vi "Edgertronic-configure_camera.vi"(3 "error in (no error)":errorcluster, 4 "Settings":T1={"Frame Rate (fps)"=1000.0, "Exposure (1/sec)"=1500.0, "Horizonal"=0, "Vertical"=0, "ISO"=500, "Duration"=1.0, "Pretrigger (%)"=50.0, "MultiShot"=1, "Subsample?"=FALSE, "Force Mono?"=FALSE, "Genlock"=enum."Off", "Overclock"=enum."Off"} {"Pretrigger (%)" min=0.0 max=100.0 step=1.0; "ISO" min=0 max=1600 step=1; "Exposure (1/sec)" min=4e-06 max=250000.0 step=1.0; "Frame Rate (fps)" min=0.1 max=25000.0 step=1.0}, 5 "URL":string="130.64.17.41") -> (0 "error out":errorcluster, 1 "Saved Settings:":T3={"Requested Genlock "="20140911165611", "Min Frame Clocks "="20140911165611", "Is Seq Clk Freq "="20140911165611", "Pretrigger Frames "="20140911165611", "Duration "="20140911165611", "Overclock "="20140911165611", "Requested Horizontal "="20140911165611", "Frames "="20140911165611", "Requested Pretrigger "="20140911165611", "Words per Frame "="20140911165611", "Buffer End "="20140911165611", "Clocks per Frame  "="20140911165611", "Requested Duration "="20140911165611", "Pretrigger "="20140911165611", "Post-trigger Frames "="20140911165611", "Vertical "="20140911165611", "Requested Vertical "="20140911165611", "Reqested Frame Rate "="20140911165611", "Frame Rate "="20140911165611", "Horizontal "="20140911165611", "Clocks per Exposure "="20140911165611", "Digital Gain "="20140911165611", "Exposure "="20140911165611", "Genlock "="20140911165611", "Analog Gain "="20140911165611", "Subsample "="20140911165611", "Requested Exposure "="20140911165611", "Iso "="20140911165611", "Requested Overclock "="20140911165611", "Requested Subsample "="20140911165611", "Requested Iso"="20140911165611", "Multishot"="20140911165611", "Requested Multishot"="20140911165611", "Monochrome"="20140911165611", "Requested mono"="20140911165611", "FPGA Temp"="20140911165611", "Is Temp"="20140911165611", "Posttrigger Duration"="20140911165611", "Pretrigger Duration"="20140911165611", "dacvrefadc"="20140911165611"})   [LabVIEW 2015]
doc: "This VI configures camera settings."
uses:
  GET/SettingsCtrl.ctl
panel:
  in  "Old ConfigCamera":T2={"Requested Genlock "="0", "Requested Horizontal (pixels)"=1110.0, "Requested Duration (seconds) "=0.5, "Requested Overclock "="0", "Requested Subsample "="0", "Reqested Force Mono"="0", "Requested Vertical (pixels)"=862.0, "Reqested Frame Rate (fps)"=14687.541250000002, "Requested Exposure (seconds)"=0.08187572500000001, "Requested Pretrigger (%)"=50.0, "Requested iso"=1038.0} {"Requested iso" min=0.0 max=1600.0 step=1.0 scale=400.0..1600.0; "Requested Pretrigger (%)" min=0.0 max=100.0 step=1.0 scale=0.0..100.0; "Requested Exposure (seconds)" min=4e-06 max=0.1 step=1.0 scale=4e-06..0.1; "Reqested Frame Rate (fps)" min=0.1 max=25000.0 step=1.0 scale=0.1..25000.0; "Requested Vertical (pixels)" min=192.0 max=1280.0 step=1.0 scale=96.0..1024.0; "Requested Duration (seconds)" min=0.0; "Requested Horizontal (pixels)" min=192.0 max=1280.0 step=1.0 scale=192.0..1280.0}
  out "POST string":string="{\"requested_horizontal\": \"733\", \"requested_vertical\": \"831\", \"requested_frame_rate\": \"1000.00\", \"requested_exposure\": \"0.002000\", \"requested_duration\": \"1.00\", \"requested_pretrigger\": \"50\", \"requested_iso\": \"500\", \"requested_subsample\": \"0\", \"requested_genlock\": \"1\", \"requested_overclock\": \"0\", \"requested_force_mono\": \"0\", \"requested_multishot_count\": \"1\"}"
  in  "Configure Camera:":T4={"Duration (sec)"=1.0, "Subsample?"=FALSE, "Force Mono?"=TRUE, "Pretrigger (%)"=50.0, "ISO"=500.0, "Horizontal"=733.0, "Vertical"=831.0, "Frame Rate (fps)"=1000.0, "Genlock"=enum."Off", "Overclock"=enum."Off", "Exposure (1/sec)"=500.0, "MultiShot"=1} {"Exposure (1/sec)" min=4e-06 max=250000.0 step=1.0 scale=10.0..250000.0; "Frame Rate (fps)" min=0.1 max=25000.0 step=1.0 scale=0.1..25000.0; "Vertical" min=192.0 max=1280.0 step=1.0 scale=96.0..1024.0; "Horizontal" min=192.0 max=1280.0 step=1.0 scale=192.0..1280.0; "ISO" min=0.0 max=1600.0 step=1.0 scale=400.0..1600.0; "Pretrigger (%)" min=0.0 max=100.0 step=1.0 scale=0.0..100.0; "Duration (sec)" min=0.0}
  # "130.64.16.195"
  # "Glossary:\nHorizontal:\t(pixels)[192-1280\t]=Width of image to capture.\nVertical:\t(pixels)[96-1024]=Height of image to capture.\nFrame Rate: (frames per second)[0.1-25000]=Number of frames to capture in every second.\nExposure:(seconds)[0.000004-0.1]=Amount of time the CMOS sensor is integrating the received light.\nDuration:(seconds)[Limited by memory]=Amount of the video to capture.\nPretrigger:(percentage)[0-100]=Amount of the video being captured is captured before the trigger event.\nIso:=sensitivity to light.\n          color:[100-400]\n          mono: [400-1600] \nSubsample: =Controls skipping every other row and column.\n          0 - off\n          1 - on\t\nForce Mono\t=Force color sensor video to be processed as monochrome. This is useful for high frame rates where the de-Bayering algorithm might add noise to the image. Note: this doesn't change the \tISO range. This feature is not implemented.\n          0 - off\n          1 - on\nGenlock:\t=Camera genlock configuration. \n          0 - off \n          1 - master =Master means the camera is generating the trigger and start-of-exposure timing signals. \n          2 - slave =Slave mean the camera is receiving those signals, via the external trigger connector, from the genlock master camera.\nOverclock: =Camera overclock configuration\n          0 - off \n          1 - A level : A is the least overclocking\n          2 - B level\n          3 - C level\n          4 - D level\t : D is the most overclocking"
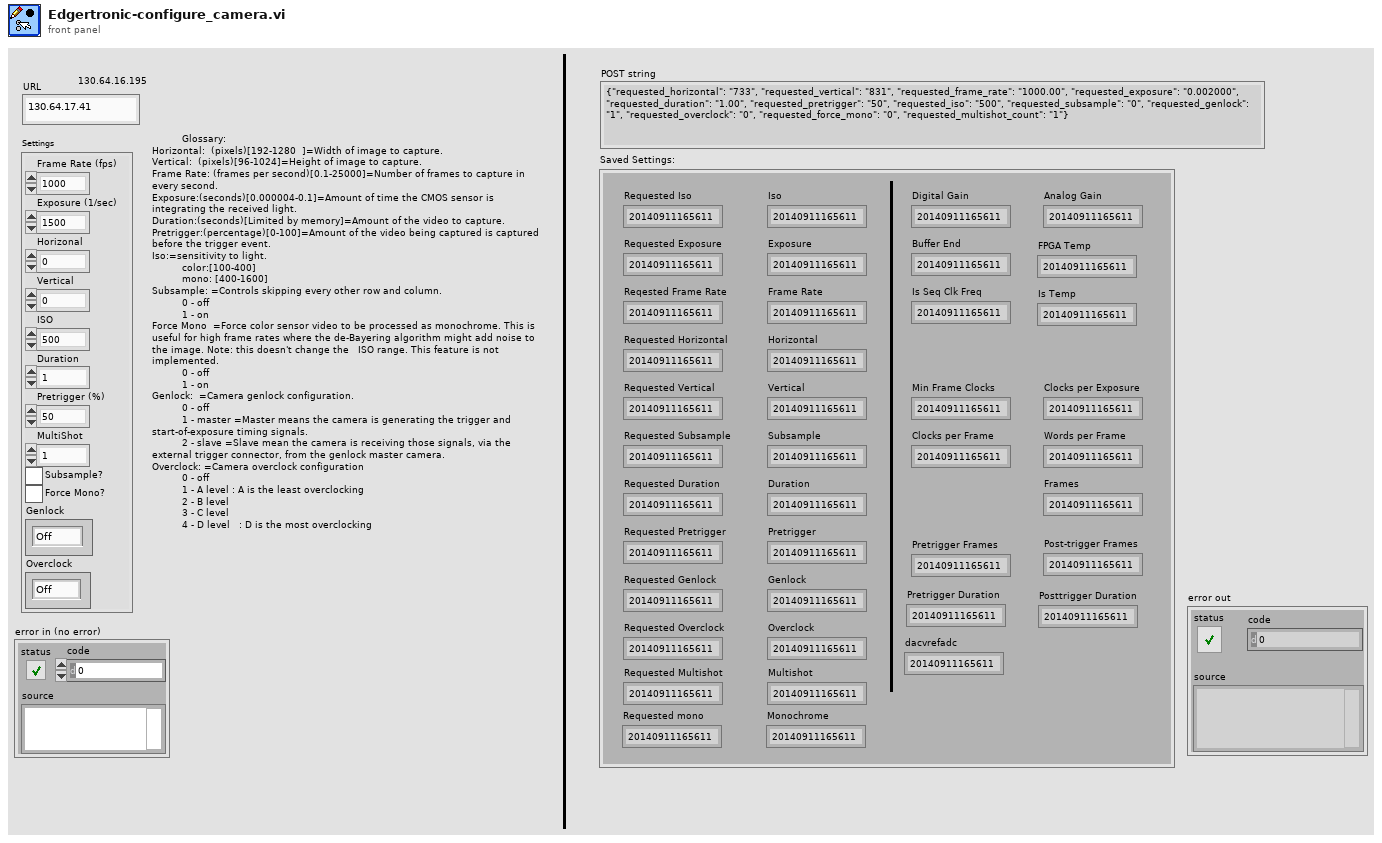
[diagram p1: front panel]
types:
  T1 = cluster{"Frame Rate (fps)":dbl, "Exposure (1/sec)":dbl, "Horizonal":u16, "Vertical":u16, "ISO":i16, "Duration":dbl, "Pretrigger (%)":dbl, "MultiShot":i16, "Subsample?":bool, "Force Mono?":bool, "Genlock":enum16{"Off", "Master", "Slave"}, "Overclock":enum16{"Off", "A level", "B Level", "C Level", "D Level"}}
  T2 = cluster{"Requested Genlock ":string, "Requested Horizontal (pixels)":dbl, "Requested Duration (seconds) ":dbl, "Requested Overclock ":string, "Requested Subsample ":string, "Reqested Force Mono":string, "Requested Vertical (pixels)":dbl, "Reqested Frame Rate (fps)":dbl, "Requested Exposure (seconds)":dbl, "Requested Pretrigger (%)":dbl, "Requested iso":dbl}
  T3 = typedef "SettingsCtrl.ctl" = cluster{"Requested Genlock ":string, "Min Frame Clocks ":string, "Is Seq Clk Freq ":string, "Pretrigger Frames ":string, "Duration ":string, "Overclock ":string, "Requested Horizontal ":string, "Frames ":string, "Requested Pretrigger ":string, "Words per Frame ":string, "Buffer End ":string, "Clocks per Frame  ":string, "Requested Duration ":string, "Pretrigger ":string, "Post-trigger Frames ":string, "Vertical ":string, "Requested Vertical ":string, "Reqested Frame Rate ":string, "Frame Rate ":string, "Horizontal ":string, "Clocks per Exposure ":string, "Digital Gain ":string, "Exposure ":string, "Genlock ":string, "Analog Gain ":string, "Subsample ":string, "Requested Exposure ":string, "Iso ":string, "Requested Overclock ":string, "Requested Subsample ":string, "Requested Iso":string, "Multishot":string, "Requested Multishot":string, "Monochrome":string, "Requested mono":string, "FPGA Temp":string, "Is Temp":string, "Posttrigger Duration":string, "Pretrigger Duration":string, "dacvrefadc":string}
  T4 = cluster{"Duration (sec)":dbl, "Subsample?":bool, "Force Mono?":bool, "Pretrigger (%)":dbl, "ISO":dbl, "Horizontal":dbl, "Vertical":dbl, "Frame Rate (fps)":dbl, "Genlock":enum16{"Off", "Master", "Slave", "External"}, "Overclock":enum16{"Off", "A level", "B Level", "C Level", "D Level"}, "Exposure (1/sec)":dbl, "MultiShot":i16}
  T5 = cluster{"Parameter":string, "Parameter 2":string, "Parameter 3":string, "Parameter 4":string, "Parameter 5":string, "Parameter 6":string, "Parameter 7":string, "Parameter 8":string, "Parameter 9":string, "Parameter 10":string, "Parameter 11":string, "Parameter 12":string}
  T6 = enum16{"Off", "A level", "B Level", "C Level", "D Level"}
  T7 = cluster{string, string, string, string, string, string, string, "output string":string, "output string":string, string, string, string}
  T8 = cluster{"Requested Genlock ":string, "Min Frame Clocks ":string, "Is Seq Clk Freq ":string, "Pretrigger Frames ":string, "Duration ":string, "Overclock ":string, "Requested Horizontal ":string, "Frames ":string, "Requested Pretrigger ":string, "Words per Frame ":string, "Buffer End ":string, "Clocks per Frame  ":string, "Requested Duration ":string, "Pretrigger ":string, "Post-trigger Frames ":string, "Vertical ":string, "Requested Vertical ":string, "Reqested Frame Rate ":string, "Frame Rate ":string, "Horizontal ":string, "Clocks per Exposure ":string, "Digital Gain ":string, "Exposure ":string, "Genlock ":string, "Analog Gain ":string, "Subsample ":string, "Requested Exposure ":string, "Iso ":string, "Requested Overclock ":string, "Requested Subsample ":string, "Requested Iso":string, "Multishot":string, "Requested Multishot":string, "Monochrome":string, "Requested mono":string, "FPGA Temp":string, "Is Temp":string, "Posttrigger Duration":string, "Pretrigger Duration":string, "dacvrefadc":string}
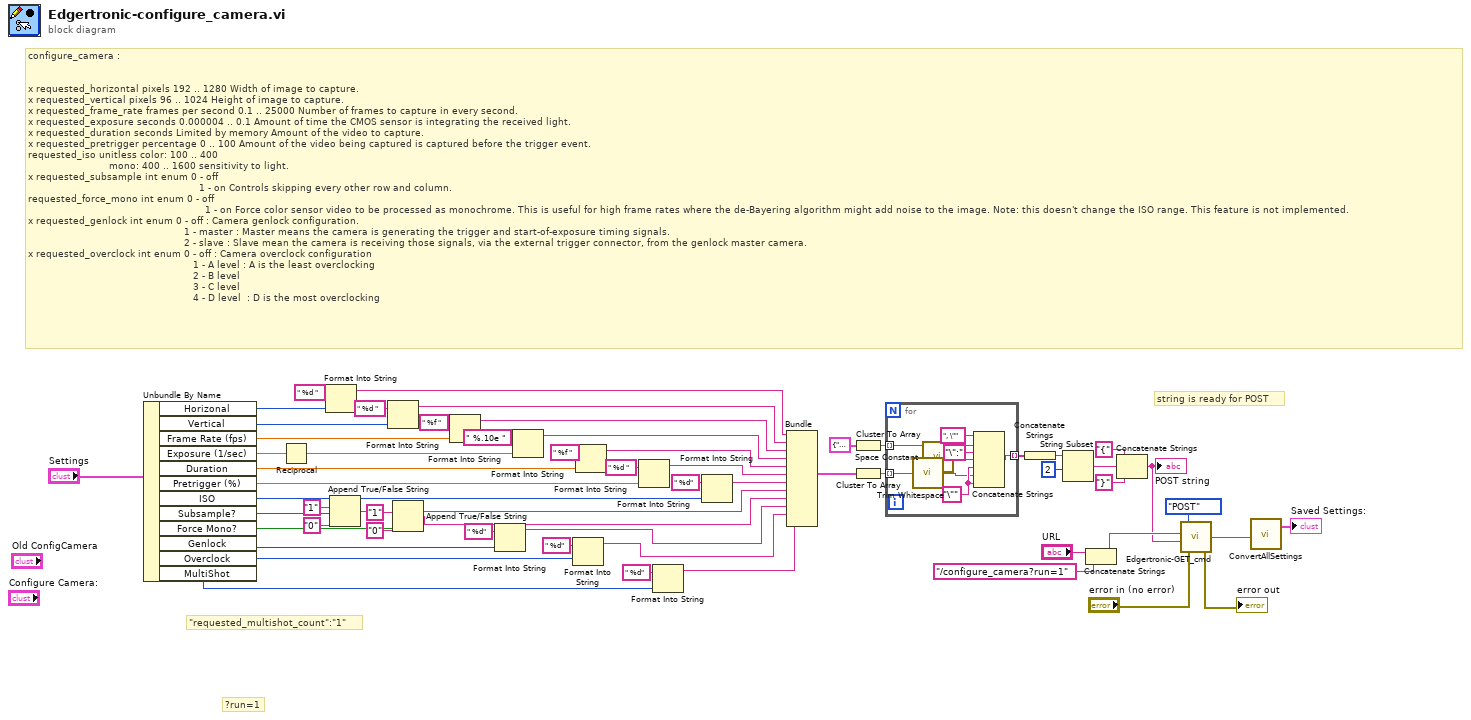
[diagram p0: block diagram]
diagram:
  # "\"requested_multishot_count\":\"1\""
  # "?run=1"
  # "string is ready for POST"
  # "configure_camera :\n\n\nx requested_horizontal\tpixels\t192 .. 1280\tWidth of image to capture.\nx requested_vertical\tpixels\t96 .. 1024\tHeight of image to capture.\nx requested_frame_rate\tframes per second\t0.1 .. 25000\tNumber of frames to capture in every second.\nx requested_exposure\tseconds\t0.000004 .. 0.1\tAmount of time the CMOS sensor is integrating the received light.\nx requested_duration\tseconds\tLimited by memory\tAmount of the video to capture.\nx requested_pretrigger\tpercentage\t0 .. 100\tAmount of the video being captured is captured before the trigger event.\nrequested_iso\tunitless\tcolor: 100 .. 400\n                           mono: 400 .. 1600\tsensitivity to light.\nx requested_subsample\tint enum\t0 - off\n                                                         1 - on\tControls skipping every other row and column.\nrequested_force_mono\tint enum\t0 - off\n                                                           1 - on\tForce color sensor video to be processed as monochrome. This is useful for high frame rates where the de-Bayering algorithm might add noise to the image. Note: this doesn't change the ISO range. This feature is not implemented.\nx requested_genlock\tint enum\t0 - off : Camera genlock configuration. \n                                                    1 - master : Master means the camera is generating the trigger and start-of-exposure timing signals. \n                                                    2 - slave : Slave mean the camera is receiving those signals, via the external trigger connector, from the genlock master camera.\nx requested_overclock int enum\t0 - off : Camera overclock configuration\n                                                       1 - A level : A is the least overclocking\n                                                       2 - B level\n                                                       3 - C level\n                                                       4 - D level\t : D is the most overclocking"
  n1 = Unbundle By Name("Settings") -> ("Horizonal"=w21:u16, "Vertical"=w20:u16, "Frame Rate (fps)"=w19:dbl, "Exposure (1/sec)"=w18:dbl, "Duration"=w17:dbl, "Pretrigger (%)"=w16:dbl, "ISO"=w15:i16, "Subsample?"=w14:bool, "Force Mono?"=w13:bool, "Genlock"=w12:enum16{"Off", "Master", "Slave"}, "Overclock"=w11:T6, "MultiShot"=w10:i16)
  n2 = Reciprocal(x=w18) -> (1/x=w25:dbl)
  n3 = Format Into String(format string=" %d ", w21) -> (resulting string=w51:string)  [unwired: 2 in, 1 out]
  n4 = Append True/False String(1:w14, 2:"0" ("false string"), 3:"1" ("true string")) -> (0:w31:string)  [unwired: 1 in]
  n5 = Format Into String(format string=" %d ", w20) -> (resulting string=w50:string)  [unwired: 2 in, 1 out]
  n6 = Append True/False String(1:w13, 2:"0" ("false string"), 3:"1" ("true string")) -> (0:w30:string)  [unwired: 1 in]
  n7 = Format Into String(format string=" %f ", w19) -> (resulting string=w49:string)  [unwired: 2 in, 1 out]
  n8 = Format Into String(format string=" %d", w12) -> (resulting string=w27:string)  [unwired: 2 in, 1 out]
  n9 = Format Into String(format string=" %.10e ", w25) -> (resulting string=w48:string)  [unwired: 2 in, 1 out]
  n10 = Format Into String(format string=" %d", w11) -> (resulting string=w26:string)  [unwired: 2 in, 1 out]
  n11 = Format Into String(format string=" %f ", w17) -> (resulting string=w47:string)  [unwired: 2 in, 1 out]
  n12 = Format Into String(format string=" %d ", w16) -> (resulting string=w46:string)  [unwired: 2 in, 1 out]
  n13 = Format Into String(format string=" %d", w10) -> (resulting string=w23:string)  [unwired: 2 in, 1 out]
  n14 = Format Into String(format string=" %d", w15) -> (resulting string=w45:string)  [unwired: 2 in, 1 out]
  n15 = Bundle(w51, w50, w49, w48, w47, w46, w45, "output string"=w31, "output string"=w30, w27, w26, w23) -> (w43:T7)  [unwired: 1 in]
  n16 = Cluster To Array(cluster=T5 {"Parameter"="requested_horizontal", "Parameter 2"="requested_vertical", "Parameter 3"="requested_frame_rate", "Parameter 4"="requested_exposure", "Parameter 5"="requested_duration", "Parameter 6"="requested_pretrigger", "Parameter 7"="requested_iso", "Parameter 8"="requested_subsample", "Parameter 9"="requested_genlock", "Parameter 10"="requested_overclock", "Parameter 11"="requested_force_mono", "Parameter 12"="requested_multishot_count"}) -> (array=w58:string[])
  n17 = Cluster To Array(cluster=w43) -> (array=w42:string[])
  n18 = for {
    tunnel: w58 -> [w64] mode=indexing
    tunnel: [w65] -> w39 mode=indexing
    tunnel: w42 -> [w63] mode=indexing
    w61 = "\"" ("string")
    n19 = call <vilib>:"Trim Whitespace.vi"("string"=w63) -> ("trimmed string"=w60:string)  [unwired: 1 in]
    n20 = call <vilib>:"Space Constant.vi"() -> ("String"=w62:string)
    n21 = Concatenate Strings(", \"" ("string"), w64, "\":" ("string"), w62, w61, w60, w61) -> (w65:string)
  }
  n22 = Concatenate Strings(w39) -> (w38:string)
  n23 = String Subset(string=w38, offset (0)=2) -> (substring=w36:string)  [unwired: 1 in]
  n24 = Concatenate Strings("URL", "/configure_camera?run=1" ("GET Command")) -> (w9:string)
  n25 = Concatenate Strings("{" ("string"), w36, "}" ("string")) -> (w5:string)
  "POST string" <- w5
  n26 = call "Edgertronic-GET_cmd.vi"("error in (no error)"="error in (no error)", "Posted Content"=w5, "URL"=w9, "Type"=enum16{"GET", "POST"}."POST") -> ("error out"=→"error out":errorcluster, "data"=w2:string)  [unwired: 1 out]
  n27 = call "ConvertAllSettings.vi"("data"=w2) -> ("Saved Settings:"=→"Saved Settings:":T8)  [unwired: 2 in]
